vi "list sub dir.vi"(8 "error in (no error)":errorcluster, 10 "path items":string[](array[string]), 11 "TCP in":refnum<k5>) -> (0 "error out":errorcluster, 2 "Array":T1[](array[typedef]), 3 "TCP out":refnum<k5>)   [LabVIEW 2020]
uses:
  ctl/7-id,name,fields.ctl
  ctl/9-id,name,path.ctl
  ctl/0-id,name.ctl
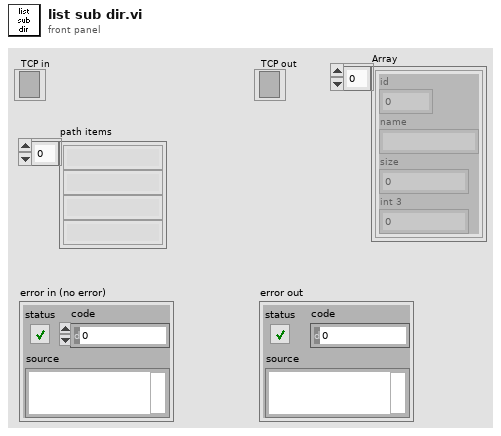
[diagram p1: front panel]
types:
  T1 = typedef "7-id,name,fields.ctl" = cluster{"id":i16, "name":string, "size":u64, "int 3":u32}
  T2 = typedef "9-id,name,path.ctl" = cluster{"id":u8, "name":string, "path":string}
  T3 = typedef "0-id,name.ctl" = cluster{"id":u8, "name":string}
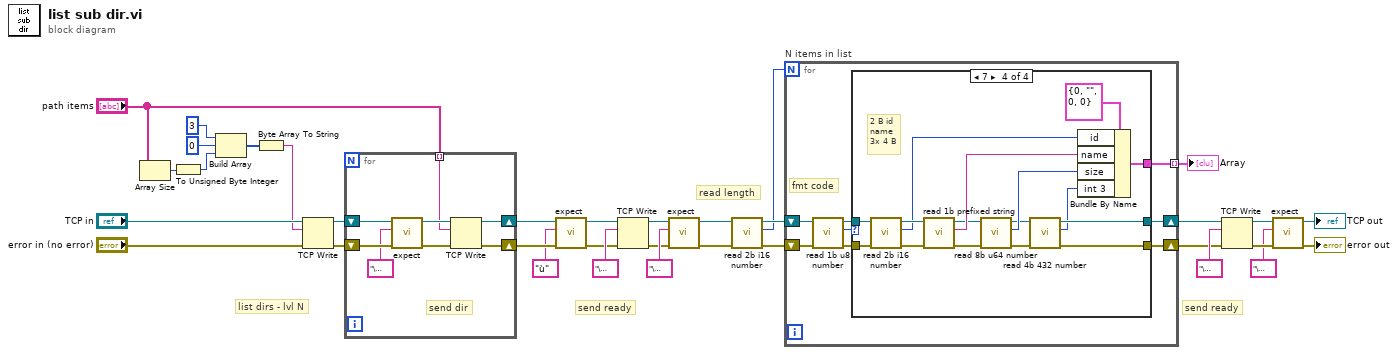
[diagram p0: block diagram]
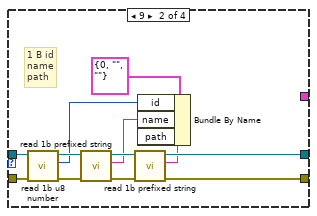
[diagram p3: hidden frame]
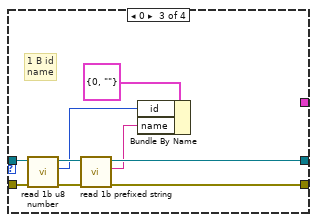
[diagram p4: hidden frame]
diagram:
  # "send ready"
  # "send ready"
  # "read length"
  # "list dirs - lvl N"
  n1 = Array Size(array="path items") -> (size(s)=w8:i32)
  n2 = To Unsigned Byte Integer(number=w8) -> (unsigned 8bit integer=w7:u8)
  n3 = Build Array(u8 3 ("element"), u8 0 ("element"), w7) -> (w4:u8[])
  n4 = Byte Array To String(unsigned byte array=w4) -> (string=w3:string)
  n5 = TCP Write(connection ID="TCP in", data in=w3, error in (no error)="error in (no error)") -> (connection ID out=w20:refnum<k5>, error out=w21:errorcluster)  [unwired: 1 in, 1 out]
  n6 = for {
    shift-right: [w41] -> w26
    shift-left: w21 -> [w39]
    shift-right: [w42] -> w27
    shift-left: w20 -> [w37]
    tunnel: "path items" -> [w35] mode=indexing
    # "send dir"
    n7 = call "expect.vi"("error in (no error)"=w39, "data expected"="\u0001" ("data in"), "TCP Network Connection in"=w37) -> ("error out"=w38:errorcluster, "TCP Network Connection out"=w40:refnum<k5>)  [unwired: 6 in, 1 out]
    n8 = TCP Write(connection ID=w40, data in=w35, error in (no error)=w38) -> (connection ID out=w42:refnum<k5>, error out=w41:errorcluster)  [unwired: 1 in, 1 out]
  }
  n9 = call "expect.vi"("error in (no error)"=w26, "data expected"="ù" ("data in"), "TCP Network Connection in"=w27) -> ("error out"=w25:errorcluster, "TCP Network Connection out"=w28:refnum<k5>)  [unwired: 6 in, 1 out]
  n10 = TCP Write(connection ID=w28, data in="\u0001", error in (no error)=w25) -> (connection ID out=w32:refnum<k5>, error out=w30:errorcluster)  [unwired: 1 in, 1 out]
  n11 = call "expect.vi"("error in (no error)"=w30, "data expected"="\u0001" ("data in"), "TCP Network Connection in"=w32) -> ("error out"=w34:errorcluster, "TCP Network Connection out"=w33:refnum<k5>)  [unwired: 6 in, 1 out]
  n12 = call "read 2b i16 number.vi"("error in (no error)"=w34, "TCP Network Connection in"=w33) -> ("error out"=w18:errorcluster, "number"=w17:i16, "TCP Network Connection out"=w19:refnum<k5>)  [unwired: 7 in]
  n13 = for "N items in list" {
    N: w17 -> [_]
    shift-right: [w45] -> w11
    shift-left: w19 -> [w50]
    shift-right: [w47] -> w12
    shift-left: w18 -> [w49]
    tunnel: [w43] -> w1 mode=indexing
    # "fmt code"
    n14 = call "read 1b u8 number.vi"("error in (no error)"=w49, "TCP Network Connection in"=w50) -> ("error out"=w48:errorcluster, "number"=w44:u8, "TCP Network Connection out"=w46:refnum<k5>)  [unwired: 7 in]
    n15 = case shown="7" w44 {
      tunnel: w48 -> [w51 w64 w73 w89]
      tunnel: [w51 w58 w68 w78] -> w47
      tunnel: w46 -> [w52 w60 w70 w86]
      tunnel: [w52 w56 w67 w76] -> w45
      tunnel: [_ _ _ w74] -> w43
      frame Default {
      }
      frame 9 {
        # "1 B id\nname\npath"
        n16 = call "read 1b u8 number.vi"("error in (no error)"=w64, "TCP Network Connection in"=w60) -> ("error out"=w61:errorcluster, "number"=w55:u8, "TCP Network Connection out"=w59:refnum<k5>)  [unwired: 7 in]
        n17 = call "read 1b prefixed string.vi"("error in (no error)"=w61, "TCP Network Connection in"=w59) -> ("error out"=w63:errorcluster, "data out"=w54:string, "TCP Network Connection out"=w57:refnum<k5>)  [unwired: 7 in]
        n18 = call "read 1b prefixed string.vi"("error in (no error)"=w63, "TCP Network Connection in"=w57) -> ("error out"=w58:errorcluster, "data out"=w53:string, "TCP Network Connection out"=w56:refnum<k5>)  [unwired: 7 in]
        n19 = Bundle By Name(cluster=T2 {"id"=0, "name"="", "path"=""} ("9 - id, len, data"), "id"=w55, "name"=w54, "path"=w53) -> ()  [unwired: 1 out]
      }
      frame 0 {
        # "1 B id\nname"
        n20 = call "read 1b u8 number.vi"("error in (no error)"=w73, "TCP Network Connection in"=w70) -> ("error out"=w71:errorcluster, "number"=w66:u8, "TCP Network Connection out"=w69:refnum<k5>)  [unwired: 7 in]
        n21 = call "read 1b prefixed string.vi"("error in (no error)"=w71, "TCP Network Connection in"=w69) -> ("error out"=w68:errorcluster, "data out"=w65:string, "TCP Network Connection out"=w67:refnum<k5>)  [unwired: 7 in]
        n22 = Bundle By Name(cluster=T3 {"id"=0, "name"=""} ("9 - id, len, data"), "id"=w66, "name"=w65) -> ()  [unwired: 1 out]
      }
      frame 7 {
        # "2 B id\nname\n3x 4 B"
        n23 = call "read 2b i16 number.vi"("error in (no error)"=w89, "TCP Network Connection in"=w86) -> ("error out"=w87:errorcluster, "number"=w83:i16, "TCP Network Connection out"=w85:refnum<k5>)  [unwired: 7 in]
        n24 = call "read 1b prefixed string.vi"("error in (no error)"=w87, "TCP Network Connection in"=w85) -> ("error out"=w84:errorcluster, "data out"=w82:string, "TCP Network Connection out"=w80:refnum<k5>)  [unwired: 7 in]
        n25 = call "read 8b u64 number.vi"("error in (no error)"=w84, "TCP Network Connection in"=w80) -> ("error out"=w81:errorcluster, "number"=w79:u64, "TCP Network Connection out"=w77:refnum<k5>)  [unwired: 7 in]
        n26 = call "read 4b 432 number.vi"("error in (no error)"=w81, "TCP Network Connection in"=w77) -> ("error out"=w78:errorcluster, "number"=w75:u32, "TCP Network Connection out"=w76:refnum<k5>)  [unwired: 7 in]
        n27 = Bundle By Name(cluster=T1 {"id"=0, "name"="", "size"=0, "int 3"=0} ("9 - id, len, data"), "id"=w83, "name"=w82, "size"=w79, "int 3"=w75) -> (w74:T1)
      }
    }
  }
  "Array" <- w1
  n28 = TCP Write(connection ID=w11, data in="\u0001", error in (no error)=w12) -> (connection ID out=w13:refnum<k5>, error out=w15:errorcluster)  [unwired: 1 in, 1 out]
  n29 = call "expect.vi"("error in (no error)"=w15, "data expected"="\u0001" ("data in"), "TCP Network Connection in"=w13) -> ("error out"=→"error out":errorcluster, "TCP Network Connection out"=→"TCP out":refnum<k5>)  [unwired: 6 in, 1 out]
